vi "SetIntakeState.vi"(11 "Input State":T1) -> ()   [LabVIEW 2017]
uses:
  StatesTypeDef.ctl
panel:
  # "input state enum"
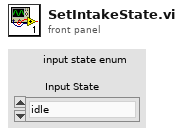
[diagram p1: front panel]
types:
  T1 = typedef "StatesTypeDef.ctl" = enum16{"idle", "lower", "raise", "feed", "spit"}
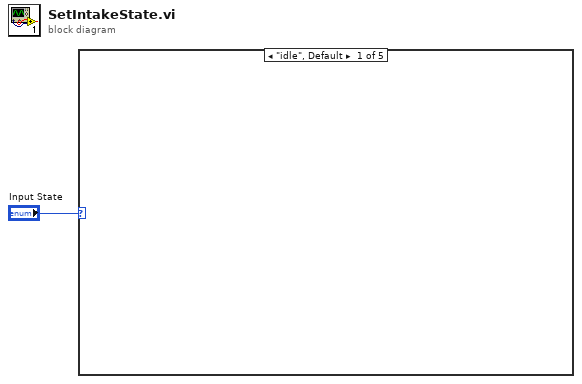
[diagram p0: block diagram]
diagram:
  n1 = case shown="\"idle\", Default" "Input State" {
    frame "idle", Default {
    }
    frame "lower" {
    }
    frame "raise" {
    }
    frame "feed" {
    }
    frame "spit" {
    }
  }
